vi "GeneratePhaseCUDAv1.vi"() -> ()   [LabVIEW 2019]
uses:
  PCIe16LabVIEWSDK/Interface.dll
panel:
  out "board":i32
  in  "Start SLM":bool
  out "Board ID":i32
  out "# of Boards":i32
  in  "SLM":bool
  in  "Z":dbl(slide) min=-100.0 max=100.0 step=1.0 scale=-100.0..100.0
  out "Delay [ms]":dbl
  out "startCuda Return":i32
  out "Init.":bool
  in  "Y":dbl(slide) min=-100.0 max=100.0 step=1.0 scale=-100.0..100.0
  in  "X":sgl(slide) min=-100 max=100 step=1 scale=-100.0..100.0
  in  "N Iterations":i32=10
  out "N Pixels":i32
  out "SLM Size":i32
  in  "CUDA":bool
  out "stopCUDA Return":i32
  out "generatePhase Return":i32
  out "Path to CUDA DLL":path
  in  "Stop":bool
  out "Phase SLM":T1(plugin-control)
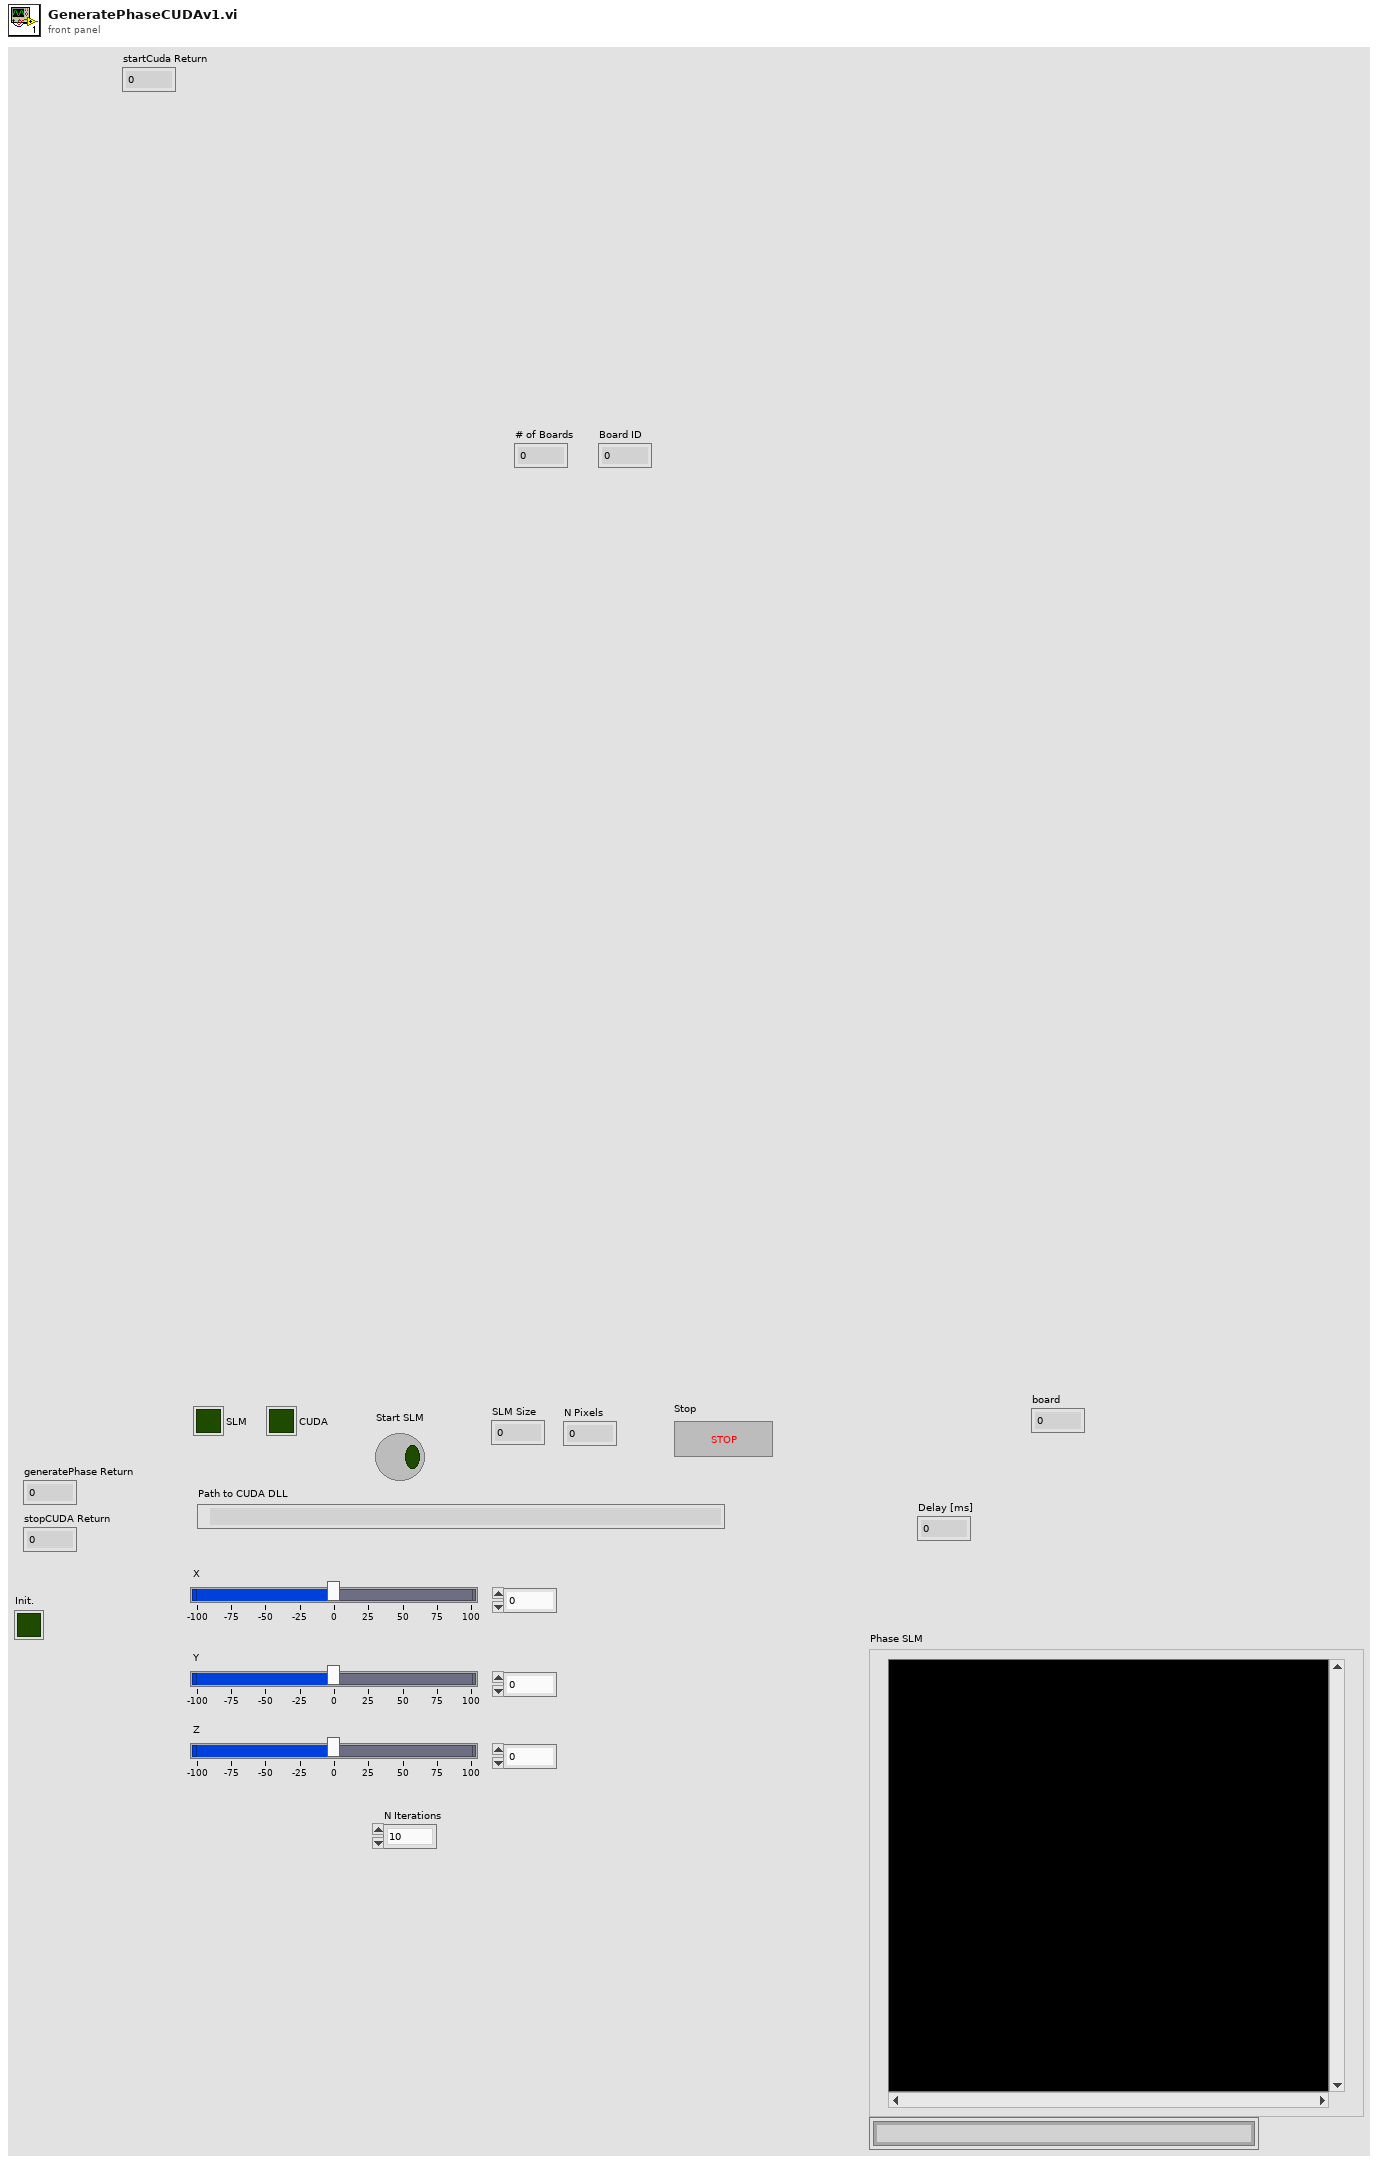
[diagram p1: front panel]
types:
  T1 = typedef "IMAQ Image.ctl" = refnum<image>
  T2 = typedef "Image Type" = u32
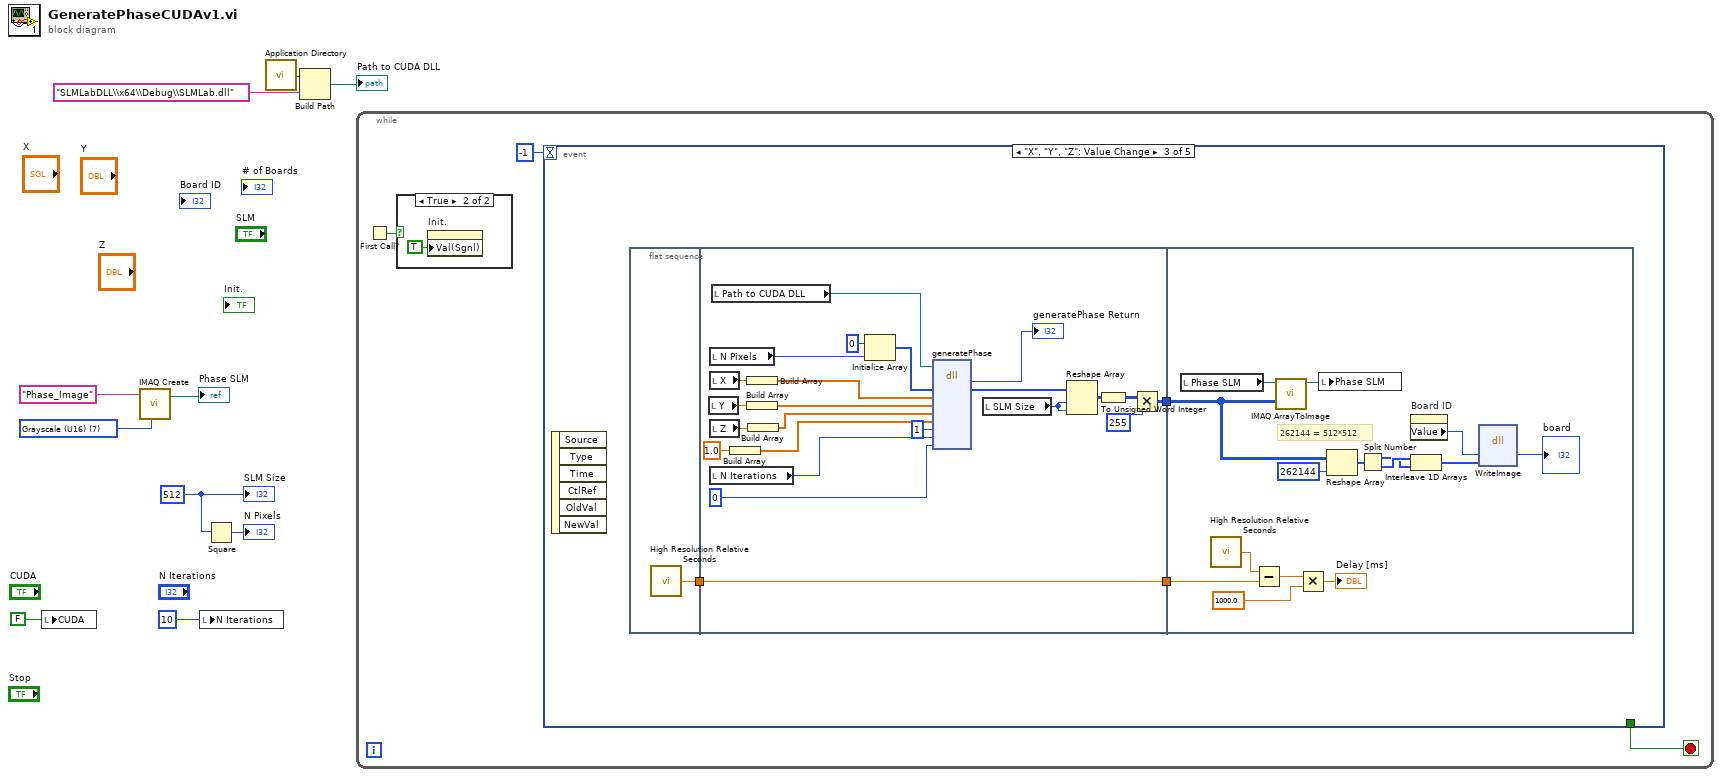
[diagram p0: block diagram]
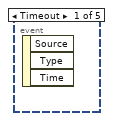
[diagram p3: hidden frame]
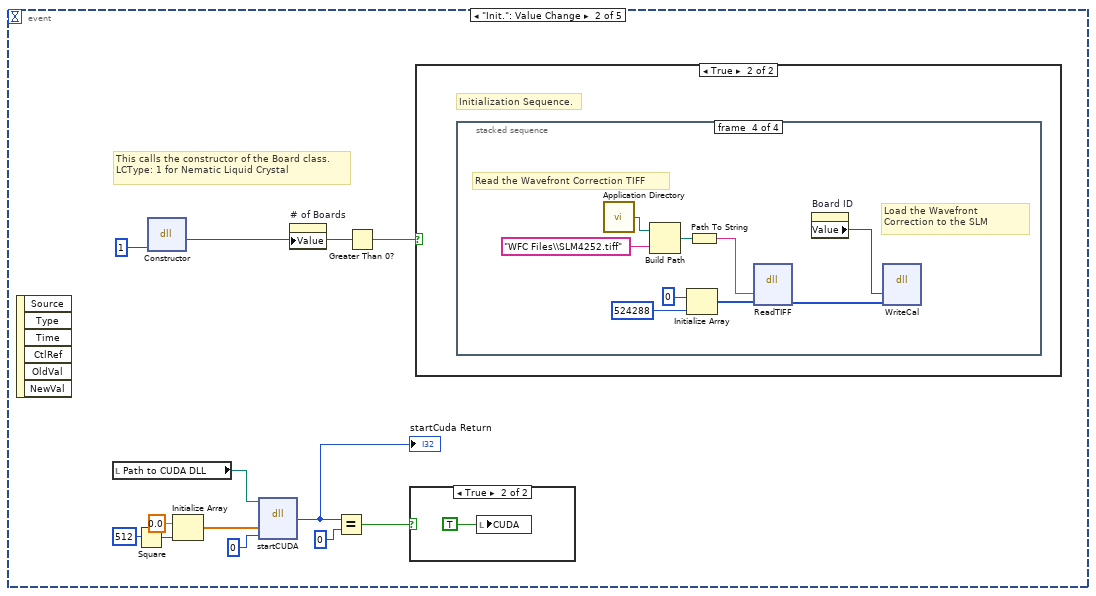
[diagram p4: hidden frame]
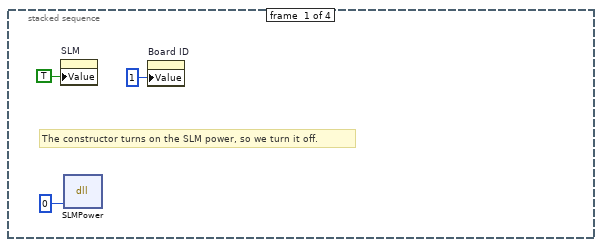
[diagram p6: hidden frame]
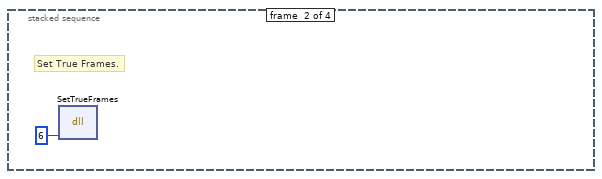
[diagram p7: hidden frame]
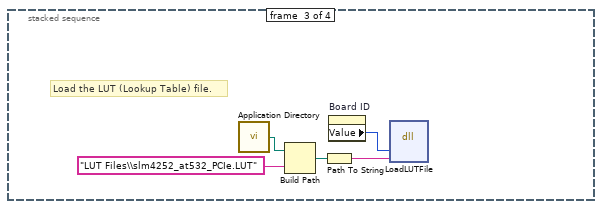
[diagram p8: hidden frame]
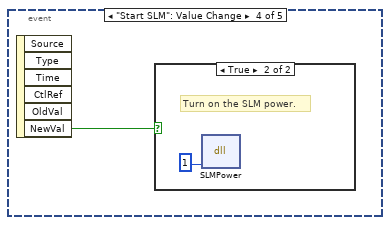
[diagram p10: hidden frame]
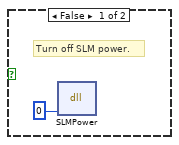
[diagram p11: hidden frame]
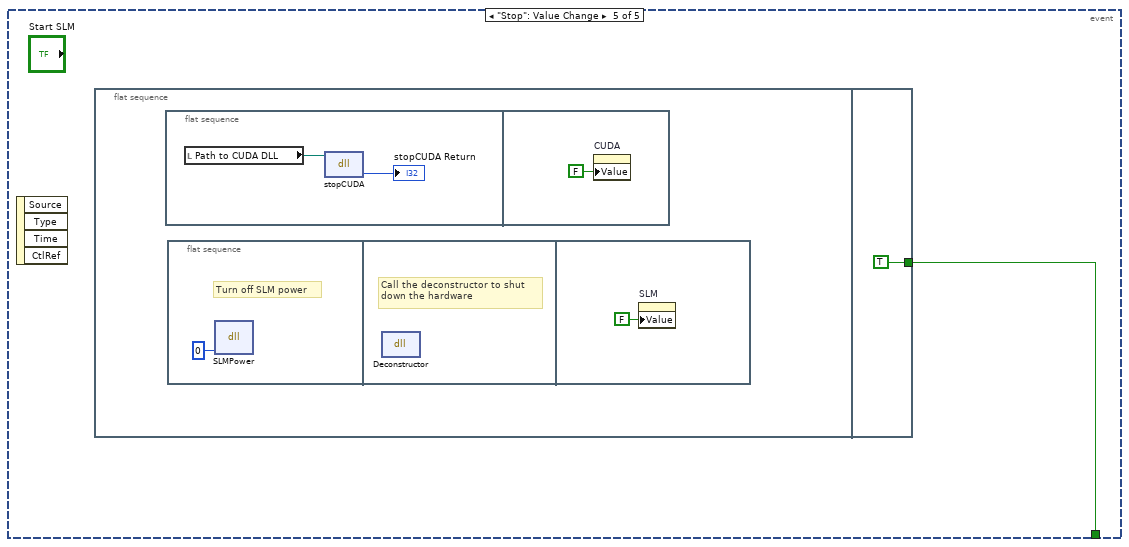
[diagram p12: hidden frame]
diagram:
  w2 = 512
  w9 = T2 7 items=["Grayscale (U8)", "Grayscale (I16)", "Grayscale (SGL)", "Complex (CSG)", "RGB (U32)", "HSL (U32)", "RGB (U64)", "Grayscale (U16)"] ("Image Type")
  n1 = local write "CUDA"(FALSE ("Update SLM")) -> ()
  n2 = call "IMAQ Create"("Image Name"="Phase_Image", "Image Type"=w9) -> ("New Image"=→"Phase SLM":T1)  [unwired: 3 in, 1 out]
  n3 = local write "N Iterations"(10) -> ()
  n4 = Square(x=w2) -> (x^2=→"N Pixels":i32)
  n5 = call <vilib>:"Application Directory.vi"() -> ("Application Directory"=w6:path)
  n6 = Build Path(base path=w6, name or relative path="SLMLabDLL\\x64\\Debug\\SLMLab.dll") -> (appended path=→"Path to CUDA DLL":path)
  n7 = while {
    stop <- w13 stop-if-true
    n8 = First Call?() -> (First Call?: T/F=w11:bool)
    n9 = case shown="True" w11 {
      frame False {
      }
      frame True {
        n10 = property on="Init." class="Bool (strict)"("Val(Sgnl)"=TRUE ("Value (Signaling)")) -> ()  [unwired: 2 in, 2 out]
      }
    }
    n11 = event shown="[2] \"X\", \"Y\", \"Z\": Value Change" {
      selector: _ -> [_ _ _ _ _]
      dyn-events: _ -> [_ _ _ _ _]
      timeout: -1 -> [_ _ _ _ _]
      tunnel: [_ _ _ _ w91] -> w13
      event Timeout {
        n12 = event-data() -> ()  [unwired: 1 in, 3 out]
      }
      event "Init.": Value Change {
        # "This calls the constructor of the Board class. LCType: 1 for Nematic Liquid Crystal"
        n13 = event-data() -> ()  [unwired: 1 in, 6 out]
        n14 = local read "Path to CUDA DLL"() -> (w24:path)
        n15 = Square(x=512 ("dimension size")) -> (x^2=w22:i32)
        n16 = dll-call lib="C:/PCIe16LabVIEWSDK/Interface.dll" fn="Constructor"("LCType"=u8 1) -> ("return type"=w17:i32)  [unwired: 4 in, 2 out]
        n17 = Initialize Array(sgl 0.0 ("element"), w22) -> (w23:sgl[])
        n18 = dll-call lib="?" fn="startCUDA"(path in=w24, "h_pSLMstart"=w23, "deviceID"=0) -> ("Rückgabetyp"=w25:i32)  [unwired: 4 in, 2 out]
        "startCuda Return" <- w25
        n19 = property on="# of Boards" class="DigNum (strict)"("Value"=w17) -> ()  [unwired: 2 in, 2 out]
        n20 = Equal?(x=w25, y=0) -> (x = y?=w26:bool)
        n21 = Greater Than 0?(x=w17) -> (x > 0?=w16:bool)
        n22 = case shown="True" w26 {
          frame False {
          }
          frame True {
            n23 = local write "CUDA"(TRUE ("Update SLM")) -> ()
          }
        }
        n24 = case shown="True" w16 {
          frame False {
          }
          frame True {
            # "Initialization Sequence."
            n25 = stacked-sequence {
              frame #0 {
                # "The constructor turns on the SLM power, so we turn it off."
                n26 = property on="SLM" class="Bool (strict)"("Value"=TRUE ("SLM")) -> ()  [unwired: 2 in, 2 out]
                n27 = dll-call lib="C:/PCIe16LabVIEWSDK/Interface.dll" fn="SLMPower"("PowerState"=0) -> ()  [unwired: 5 in, 2 out]
                n28 = property on="Board ID" class="DigNum (strict)"("Value"=1 ("Board Number")) -> ()  [unwired: 2 in, 2 out]
              }
              frame #1 {
                # "Set True Frames."
                n29 = dll-call lib="C:/PCIe16LabVIEWSDK/Interface.dll" fn="SetTrueFrames"("TrueFrames"=6) -> ()  [unwired: 5 in, 2 out]
              }
              frame #2 {
                # "Load the LUT (Lookup Table) file."
                n30 = call <vilib>:"Application Directory.vi"() -> ("Application Directory"=w33:path)
                n31 = Build Path(base path=w33, name or relative path="LUT Files\\slm4252_at532_PCIe.LUT") -> (appended path=w34:path)
                n32 = Path To String(path=w34) -> (string=w31:string)
                n33 = property on="Board ID" class="DigNum (strict)"() -> ("Value"=w35:i32)  [unwired: 2 in, 2 out]
                n34 = dll-call lib="C:/PCIe16LabVIEWSDK/Interface.dll" fn="LoadLUTFile"("board"=w35, "LUTPath"=w31) -> ()  [unwired: 6 in, 2 out]
              }
              frame #3 {
                # "Read the Wavefront Correction TIFF"
                # "Load the Wavefront Correction to the SLM"
                n35 = call <vilib>:"Application Directory.vi"() -> ("Application Directory"=w41:path)
                n36 = Build Path(base path=w41, name or relative path="WFC Files\\SLM4252.tiff") -> (appended path=w42:path)
                n37 = Initialize Array(u8 0, 524288) -> (w36:u8[])
                n38 = Path To String(path=w42) -> (string=w39:string)
                n39 = dll-call lib="C:/PCIe16LabVIEWSDK/Interface.dll" fn="ReadTIFF"("TiffPath"=w39, "Image"=w36) -> ("Image"=w44:u8[])  [unwired: 5 in, 2 out]
                n40 = property on="Board ID" class="DigNum (strict)"() -> ("Value"=w43:i32)  [unwired: 2 in, 2 out]
                n41 = dll-call lib="C:/PCIe16LabVIEWSDK/Interface.dll" fn="WriteCal"("board"=w43, "Image"=w44) -> ()  [unwired: 6 in, 2 out]
              }
            }
          }
        }
      }
      event "X", "Y", "Z": Value Change {
        n42 = event-data() -> ()  [unwired: 1 in, 6 out]
        n43 = flat-sequence {
          tunnel: [w49] -> w47
          tunnel: [w55] -> w48
          tunnel: w47 -> [w55]
          tunnel: [w53] -> w46
          tunnel: w48 -> [w87]
          tunnel: w46 -> [w74]
          frame #0 {
            n44 = call <vilib>:"High Resolution Relative Seconds.vi"() -> ("relative seconds"=w49:dbl)
          }
          frame #1 {
            n45 = local read "Y"() -> (w69:dbl)
            n46 = local read "N Pixels"() -> (w64:i32)
            n47 = local read "X"() -> (w67:sgl)
            n48 = local read "Z"() -> (w54:dbl)
            n49 = local read "N Iterations"() -> (w66:i32)
            n50 = local read "Path to CUDA DLL"() -> (w63:path)
            n51 = Build Array(1.0 ("element")) -> (w72:dbl[])
            n52 = Build Array(w67) -> (w68:sgl[])
            n53 = Build Array(w69) -> (w70:dbl[])
            n54 = Build Array(w54) -> (w71:dbl[])
            n55 = Initialize Array(u16 0 ("element"), w64) -> (w62:u16[])
            n56 = dll-call lib="?" fn="generatePhase"(path in=w63, "h_pSLM_uint16"=w62, "x_spots"=w68, "y_spots"=w70, "z_spots"=w71, "I_spots"=w72, "N_spots"=1, "N_interations"=w66, "method"=0) -> ("Return Value"=→"generatePhase Return":i32, "h_pSLM_uint16"=w61:u8[])  [unwired: 9 in, 2 out]
            n57 = local read "SLM Size"() -> (w65:i32)
            n58 = Reshape Array(w61, w65, w65) -> (w52:u8[][])
            n59 = To Unsigned Word Integer(number=w52) -> (unsigned 16bit integer=w51:u16[][])
            n60 = Multiply(x=w51, y=u16 255) -> (x*y=w53:u16[][])
          }
          frame #2 {
            # "262144 = 512*512"
            n61 = local read "Phase SLM"() -> (w81:T1)
            n62 = call <vilib>:"High Resolution Relative Seconds.vi"() -> ("relative seconds"=w86:dbl)
            n63 = Subtract(x=w86, y=w87) -> (x-y=w85:dbl)
            n64 = call "IMAQ ArrayToImage"("Image Pixels (U16)"=w74, "Image"=w81) -> ("Image Out"=w82:T1)  [unwired: 8 in, 1 out]
            n65 = Multiply(x=w85, y=1000.0) -> (x*y=→"Delay [ms]":dbl)
            n66 = local write "Phase SLM"(w82) -> ()
            n67 = Reshape Array(w74, 262144 ("dimension size")) -> (w79:u16[])
            n68 = Split Number(x=w79) -> (hi(x)=w76:u8[], lo(x)=w77:u8[])
            n69 = property on="Board ID" class="DigNum (strict)"() -> ("Value"=w80:i32)  [unwired: 2 in, 2 out]
            n70 = Interleave 1D Arrays(w77, w76) -> (w78:u8[])
            n71 = dll-call lib="C:/PCIe16LabVIEWSDK/Interface.dll" fn="WriteImage"("board"=w80, "Image"=w78) -> ("board"=→"board":i32)  [unwired: 5 in, 2 out]
          }
        }
      }
      event "Start SLM": Value Change {
        n72 = event-data() -> ("NewVal"=w88:bool)  [unwired: 1 in, 5 out]
        n73 = case shown="True" w88 {
          frame False {
            # "Turn off SLM power."
            n74 = dll-call lib="C:/PCIe16LabVIEWSDK/Interface.dll" fn="SLMPower"("PowerState"=0) -> ()  [unwired: 5 in, 2 out]
          }
          frame True {
            # "Turn on the SLM power."
            n75 = dll-call lib="C:/PCIe16LabVIEWSDK/Interface.dll" fn="SLMPower"("PowerState"=1) -> ()  [unwired: 5 in, 2 out]
          }
        }
      }
      event "Stop": Value Change {
        n76 = event-data() -> ()  [unwired: 1 in, 4 out]
        n77 = flat-sequence {
          tunnel: [TRUE] -> w91
          frame #0 {
            n78 = flat-sequence {
              frame #0 {
                n79 = local read "Path to CUDA DLL"() -> (w92:path)
                n80 = dll-call lib="?" fn="stopCUDA"(path in=w92) -> ("Return Value"=→"stopCUDA Return":i32)  [unwired: 2 in, 2 out]
              }
              frame #1 {
                n81 = property on="CUDA" class="Bool (strict)"("Value"=FALSE ("SLM")) -> ()  [unwired: 2 in, 2 out]
              }
            }
            n82 = flat-sequence {
              frame #0 {
                # "Turn off SLM power"
                n83 = dll-call lib="C:/PCIe16LabVIEWSDK/Interface.dll" fn="SLMPower"("PowerState"=0) -> ()  [unwired: 5 in, 2 out]
              }
              frame #1 {
                # "Call the deconstructor to shut \ndown the hardware"
                n84 = dll-call lib="C:/PCIe16LabVIEWSDK/Interface.dll" fn="Deconstructor"() -> ()  [unwired: 4 in, 2 out]
              }
              frame #2 {
                n85 = property on="SLM" class="Bool (strict)"("Value"=FALSE ("SLM")) -> ()  [unwired: 2 in, 2 out]
              }
            }
          }
          frame #1 {
          }
        }
      }
    }
  }
  "SLM Size" <- w2
